vi "process error.vi"(10 "Error Object":refnum<class>, 11 "Template in":refnum<class "Template.lvclass">) -> ()   [LabVIEW 2020, in "Template.lvlib" / "Template.lvclass"]
uses:
  Template.lvclass
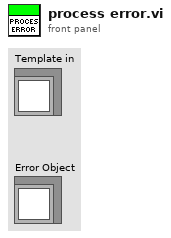
[diagram p1: front panel]
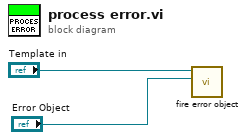
[diagram p0: block diagram]
diagram:
  n1 = call "fire error object.vi"("Error in"="Error Object", "Template in"="Template in") -> ()  [unwired: 10 in]
